vi "load_specification_file.vi"(9 "LUA Specification File":path, 10 "Parameters Tree":refnum<vi>, 11 "Digital in":refnum<vi>) -> ()   [LabVIEW 2019]
uses:
  Biogas_LabView_Wrapper/lib/libBioGasLabViewWrapper.so
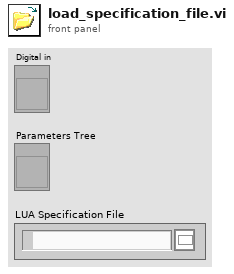
[diagram p1: front panel]
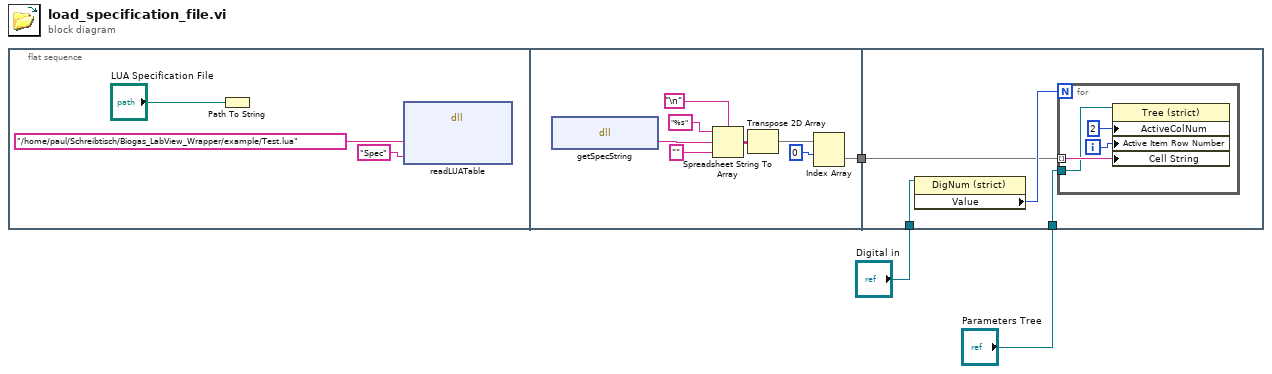
[diagram p0: block diagram]
diagram:
  n1 = flat-sequence {
    tunnel: [w8] -> w3
    tunnel: w3 -> [w17]
    tunnel: "Parameters Tree" -> [w16]
    tunnel: "Digital in" -> [w15]
    frame #0 {
      n2 = Path To String(path="LUA Specification File") -> ()  [unwired: 1 out]
      n3 = dll-call lib="home/paul/Schreibtisch/Biogas_LabView_Wrapper/lib/libBioGasLabViewWrapper.so" fn="readLUATable"("filename"="/home/paul/Schreibtisch/Biogas_LabView_Wrapper/example/Test.lua", "vali_or_spec"="Spec" ("spec_filename")) -> ()  [unwired: 6 in, 2 out]
    }
    frame #1 {
      n4 = dll-call lib="home/paul/Schreibtisch/Biogas_LabView_Wrapper/lib/libBioGasLabViewWrapper.so" fn="getSpecString"() -> ("return type"=w12:string)  [unwired: 3 in, 2 out]
      n5 = Spreadsheet String To Array(delimiter (Tab)="\n", format string="%s", spreadsheet string=w12, array type (2D Dbl)="") -> (array=w13:string[][])
      n6 = Transpose 2D Array(2D array=w13) -> (transposed array=w14:string[][])
      n7 = Index Array(array=w14, index (row)=0) -> (element=w8:string[])  [unwired: 1 in]
    }
    frame #2 {
      n8 = property class="DigNum (strict)"(reference=w15) -> ("Value"=w18:i32)  [unwired: 1 in, 2 out]
      n9 = for {
        N: w18 -> [_]
        tunnel: w17 -> [w20] mode=indexing
        tunnel: w16 -> [w19]
        i -> [w21]
        n10 = property on="Property Node" class="Tree (strict)"(reference=w19, "ActiveColNum"=2 ("Active Cell:Active Column Number"), "Active Item Row Number"=w21, "Cell String"=w20) -> ()  [unwired: 1 in, 2 out]
      }
    }
  }
